vi "start angle vi.vi"(11 "X":dbl=0.8 format="%#_13g") -> (3 "theta0":dbl)   [LabVIEW 2014]
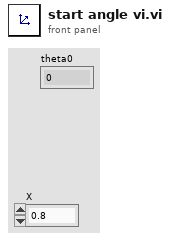
[diagram p1: front panel]
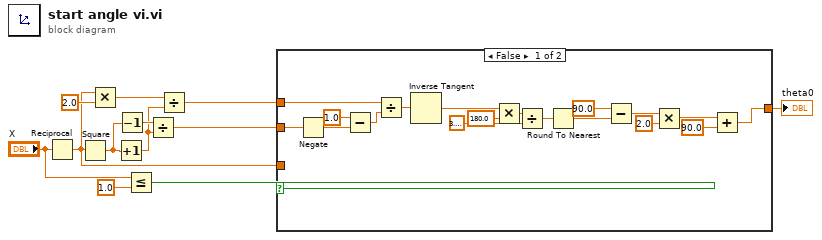
[diagram p0: block diagram]
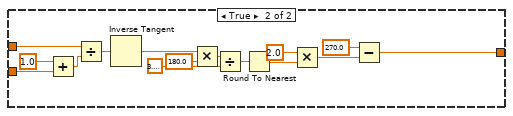
[diagram p2: hidden frame]
diagram:
  n1 = Reciprocal(x="X") -> (1/x=w2:dbl)
  n2 = Square(x=w2) -> (x^2=w12:dbl)
  n3 = Multiply(x=w2, y=2.0) -> (x*y=w9:dbl)
  n4 = Increment(x=w12) -> (x+1=w8:dbl)
  n5 = Decrement(x=w12) -> (x-1=w11:dbl)
  n6 = Less Or Equal?(x="X", y=1.0) -> (x <= y?=w5:bool)
  n7 = Divide(x=w11, y=w8) -> (x/y=w4:dbl)
  n8 = Divide(x=w9, y=w8) -> (x/y=w3:dbl)
  n9 = case shown="False" w5 {
    tunnel: w4 -> [w24 w37]
    tunnel: w3 -> [w25 w36]
    tunnel: [w13 w31] -> w1
    tunnel: w2 -> [_ _]
    frame False {
      n10 = Negate(x=w24) -> (-x=w21:dbl)
      n11 = Subtract(x=1.0, y=w21) -> (x-y=w22:dbl)
      n12 = Divide(x=w25, y=w22) -> (x/y=w26:dbl)
      n13 = Inverse Tangent(1:w26) -> (0:w30:dbl)
      n14 = Multiply(x=w30, y=180.0) -> (x*y=w28:dbl)
      n15 = Divide(x=w28, y=3.141592653589793) -> (x/y=w20:dbl)
      n16 = Round To Nearest(number=w20) -> (nearest integer value=w16:dbl)
      n17 = Subtract(x=90.0, y=w16) -> (x-y=w18:dbl)
      n18 = Multiply(x=w18, y=2.0) -> (x*y=w15:dbl)
      n19 = Add(x=w15, y=90.0) -> (x+y=w13:dbl)
    }
    frame True {
      n20 = Add(x=1.0, y=w37) -> (x+y=w39:dbl)
      n21 = Divide(x=w36, y=w39) -> (x/y=w41:dbl)
      n22 = Inverse Tangent(1:w41) -> (0:w45:dbl)
      n23 = Multiply(x=w45, y=180.0) -> (x*y=w43:dbl)
      n24 = Divide(x=w43, y=3.141592653589793) -> (x/y=w40:dbl)
      n25 = Round To Nearest(number=w40) -> (nearest integer value=w34:dbl)
      n26 = Multiply(x=2.0, y=w34) -> (x*y=w32:dbl)
      n27 = Subtract(x=270.0, y=w32) -> (x-y=w31:dbl)
    }
  }
  "theta0" <- w1
